vi "Edit.vi"(7 "Action":enum16{"Add", "Insert", "Modify", "Delete"}(ring), 8 "error in (no error)":errorcluster, 10 "Step":i32, 11 "Macro in":refnum<class "Macro.lvclass">) -> (0 "error out":errorcluster, 3 "Macro out":refnum<class "Macro.lvclass">)   [LabVIEW 2020, in "MacroAssert.lvlib" / "Macro.lvclass"]
uses:
  Macro.lvclass
  Macro.lvclass/Macro.ctl
  MacroAssert.lvlib
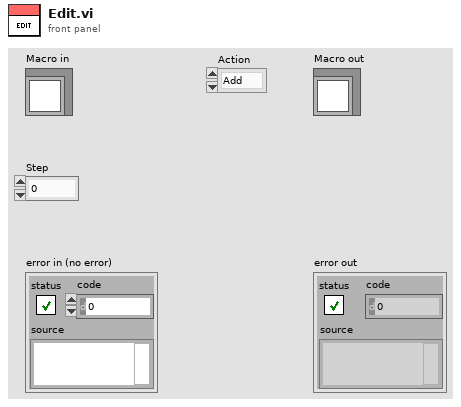
[diagram p1: front panel]
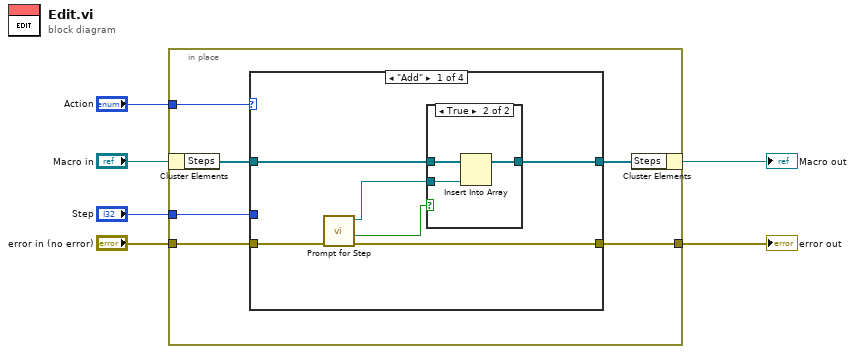
[diagram p0: block diagram]
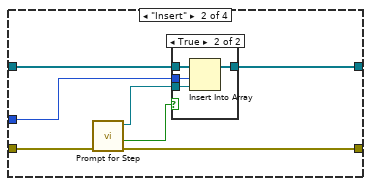
[diagram p3: hidden frame]
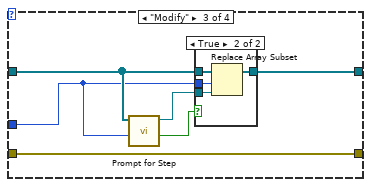
[diagram p5: hidden frame]
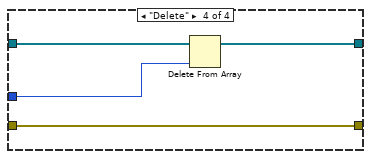
[diagram p7: hidden frame]
diagram:
  n1 = in-place {
    in-place-border: "Action" -> [w12]
    in-place-border: "Step" -> [w11]
    in-place-border: "error in (no error)" -> [w8]
    in-place-border: [w7] -> w1
    n2 = in-place-cluster #1("Macro in") -> ("Steps"=w10:refnum<class "Step.lvclass">[])
    n3 = case shown="\"Add\"" w12 {
      tunnel: w10 -> [w15 w29 w40 w49]
      tunnel: [w17 w28 w39 w48] -> w9
      tunnel: w11 -> [_ w25 w37 w47]
      tunnel: w8 -> [w14 w24 w35 w46]
      tunnel: [w13 w23 w35 w46] -> w7
      frame "Add" {
        n4 = call "Prompt for Step.vi"("error in (no error)"=w14) -> ("error out"=w13:errorcluster, "OK?"=w16:bool, "Step"=w18:refnum<class "Step.lvclass">)  [unwired: 8 in]
        n5 = case shown="True" w16 {
          tunnel: w18 -> [_ w22]
          tunnel: w15 -> [w19 w21]
          tunnel: [w19 w20] -> w17
          frame False {
          }
          frame True {
            n6 = Insert Into Array(array=w21, new element=w22) -> (w20:refnum<class "Step.lvclass">[])  [unwired: 1 in]
          }
        }
      }
      frame "Insert" {
        n7 = call "Prompt for Step.vi"("error in (no error)"=w24) -> ("error out"=w23:errorcluster, "OK?"=w26:bool, "Step"=w27:refnum<class "Step.lvclass">)  [unwired: 8 in]
        n8 = case shown="True" w26 {
          tunnel: w25 -> [_ w34]
          tunnel: w27 -> [_ w33]
          tunnel: w29 -> [w30 w32]
          tunnel: [w30 w31] -> w28
          frame False {
          }
          frame True {
            n9 = Insert Into Array(array=w32, index=w34, new element=w33) -> (w31:refnum<class "Step.lvclass">[])
          }
        }
      }
      frame "Modify" {
        n10 = call "Prompt for Step.vi"("Index"=w37, "Steps"=w40) -> ("OK?"=w38:bool, "Step"=w36:refnum<class "Step.lvclass">)  [unwired: 7 in, 1 out]
        n11 = case shown="True" w38 {
          tunnel: w37 -> [_ w45]
          tunnel: w36 -> [_ w44]
          tunnel: [w41 w43] -> w39
          tunnel: w40 -> [w41 w42]
          frame False {
          }
          frame True {
            n12 = Replace Array Subset(array=w42, new element=w44, index=w45) -> (w43:refnum<class "Step.lvclass">[])
          }
        }
      }
      frame "Delete" {
        n13 = Delete From Array(array=w49, index=w47) -> (array with subset deleted=w48:refnum<class "Step.lvclass">[])  [unwired: 1 in, 1 out]
      }
    }
    n14 = in-place-cluster #1("Steps"=w9) -> (→"Macro out":refnum<class "Macro.lvclass">)
  }
  "error out" <- w1
